vi "总磷总氮通讯.vi"() -> ()   [LabVIEW 2016, in "斯坦道总磷总氮.lvlib"]
uses:
  <vilib>/Plasmionique/MB Master/MB_Master_TCP/MB_Master_TCP.lvclass
  D:/Program Files (x86)/National Instruments/LabVIEW 2016/vi.lib/Plasmionique/MB Master/MB_Master/MB_Master.lvclass
  <vilib>/NI/Modbus Library/API/Wrapper/Create TCP Slave.vi
  <vilib>/Utility/config.llb/Write Key (Boolean).vi
  <vilib>/Utility/config.llb/Write Key (String).vi
  <vilib>/Plasmionique/MB Master/MB_Master/MB_Master.lvclass
  <vilib>/NI/Modbus Library/API/slave/Modbus Slave.lvclass
  <vilib>/Utility/config.llb/NI_LVConfig.lvlib
  <vilib>/Plasmionique/MB Master/MB Master.lvlib
  <vilib>/NI/Modbus Library/API/Wrapper/API Main.lvlib
panel:
  out "总氮测量数据区":u16[](array[numeric])
  out "总氮状态告警区":u16[](array[numeric])
  out "总磷状态告警区":u16[](array[numeric])
  out "总磷测量数据区":u16[](array[numeric])
  out "序列号":string
  out "状态告警区":T1
  out "测量数据区":T2 {"单位" items=["ug/L", "mg/L", "ppm", "mg/m3", "cm", "ppb", "ug/m3", "%", "nmol/mol", "umol/mol", "MPN/L", "MPN/100ml", "ng/m3", "NTU", "无量纲", "ms/cm", "us/cm", "℃", "mV", "万个/L"]}
  out "status":bool
  out "关键参数区":T3
  in  "读关键参数区":bool
  in  "读状态告警区":bool
  in  "读测量数据区":bool
  in  "站号":u16(ring) items=["总磷"=1, "氨氮"=3]
  in  "停止":bool
  in  "启动":bool
  in  "控制命令":u16(ring) items=["启动测量"=1, "标样核查"=2, "零点核查"=3, "跨度核查"=4, "空白测试"=5, "平行样测试"=6, "加标回收"=7, "空白校准"=8, "标样校准"=9, "初始化（清洗）"=10, "停止测试"=11, "仪器重启"=12, "校时"=13, "模式设置"=14, "测量间隔设置"=15]
  in  "控制命令参数":u16[](array[numeric]) format="%04xH"
  in  "VISA Resource":refnum<visa-resource-name>
  in  "启用模块":bool
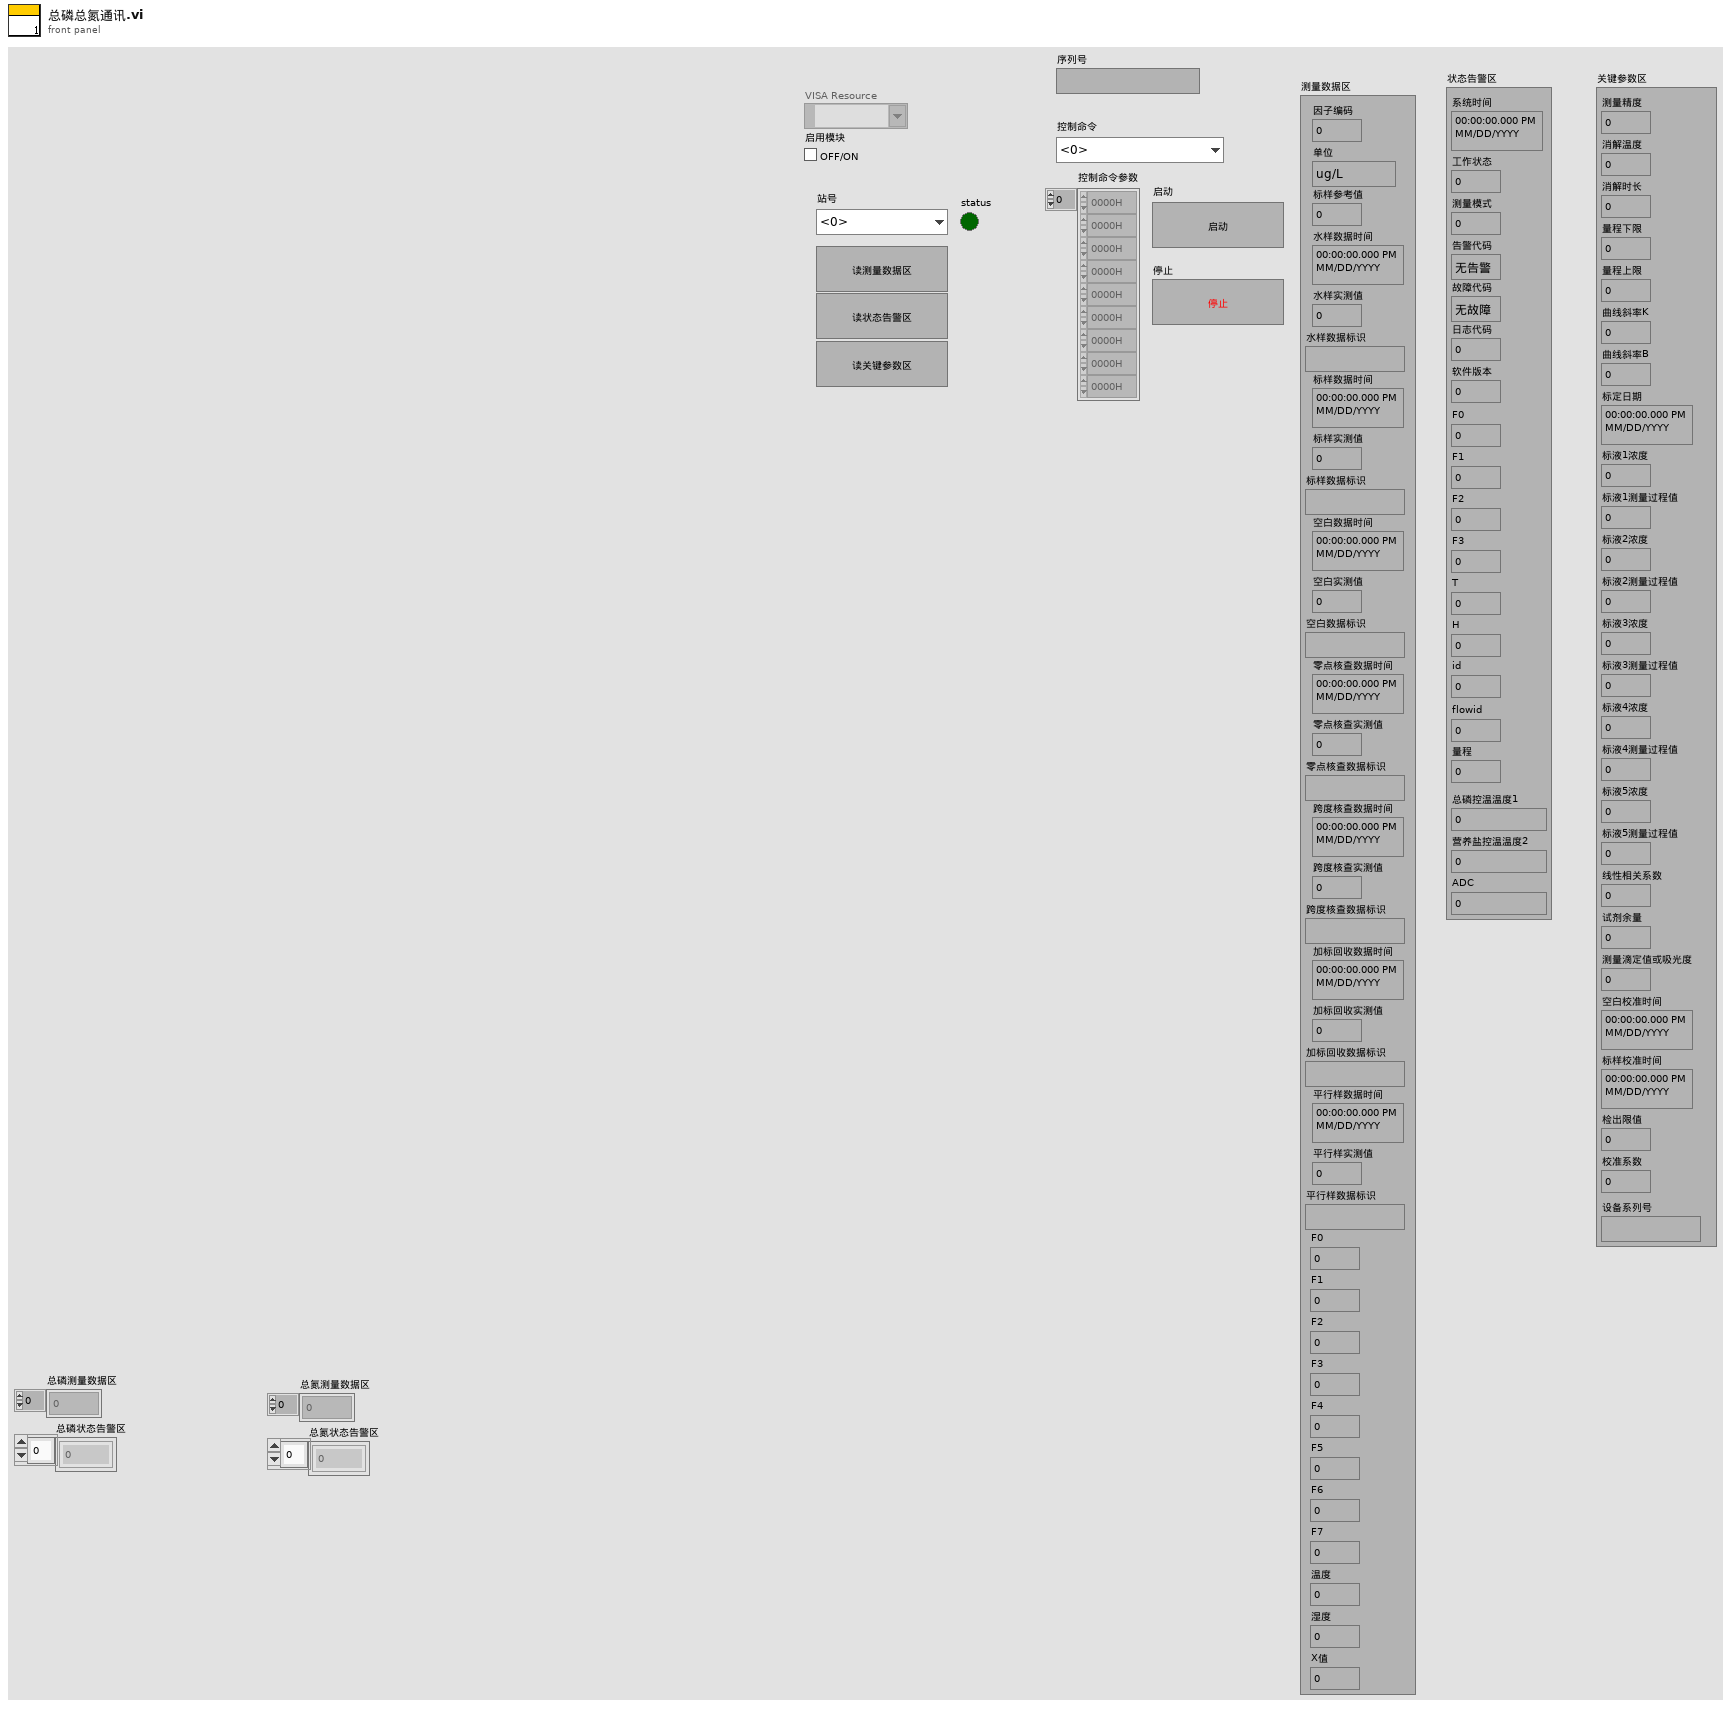
[diagram p1: front panel]
types:
  T1 = cluster{"系统时间":timestamp, "工作状态":u16, "测量模式":u16, "告警代码":enum16{"无告警", "缺试剂告警", "缺水样告警", "缺蒸馏水告警", "缺标液告警", "仪表漏液告警", "标定异常告警", "超量程告警", "加热异常", "低试剂预警", "超上限告警", "超下限告警", "仪表内部其他异常", "滴定异常告警", "电极异常告警", "量程切换告警", "参数设置告警", "PH电极电位异常", "电导率电极异常", "浊度光度异常", "溶解氧电极异常", "溶解氧光强异常", "温度异常告警", "PH异常告警", "溶解氧异常告警", "电导率异常告警", "浊度异常告警", "叶绿素异常告警", "藻密度异常告警", "蓝绿藻异常告警", "ORP异常告警", "氨氮异常告警", "清洁刷异常告警", "SD卡异常告警", "蓝牙异常告警", "Wifi异常告警", "流程异常告警"}, "故障代码":enum16{"无故障", "电机故障", "温度故障", "通讯故障", "滴定故障"}, "日志代码":u16, "软件版本":u16, "F0":sgl, "F1":sgl, "F2":sgl, "F3":sgl, "T":sgl, "H":sgl, "id":u16, "flowid":u16, "量程":u16, "总磷控温温度1":sgl, "营养盐控温温度2":sgl, "ADC":sgl}
  T2 = cluster{"因子编码":u32, "单位":u16, "标样参考值":sgl, "水样数据时间":timestamp, "水样实测值":sgl, "水样数据标识":string, "标样数据时间":timestamp, "标样实测值":sgl, "标样数据标识":string, "空白数据时间":timestamp, "空白实测值":sgl, "空白数据标识":string, "零点核查数据时间":timestamp, "零点核查实测值":sgl, "零点核查数据标识":string, "跨度核查数据时间":timestamp, "跨度核查实测值":sgl, "跨度核查数据标识":string, "加标回收数据时间":timestamp, "加标回收实测值":sgl, "加标回收数据标识":string, "平行样数据时间":timestamp, "平行样实测值":sgl, "平行样数据标识":string, "F0":sgl, "F1":sgl, "F2":sgl, "F3":sgl, "F4":sgl, "F5":sgl, "F6":sgl, "F7":sgl, "温度":sgl, "湿度":sgl, "X值":sgl}
  T3 = cluster{"测量精度":u16, "消解温度":u16, "消解时长":u16, "量程下限":sgl, "量程上限":sgl, "曲线斜率K":sgl, "曲线斜率B":sgl, "标定日期":timestamp, "标液1浓度":sgl, "标液1测量过程值":sgl, "标液2浓度":sgl, "标液2测量过程值":sgl, "标液3浓度":sgl, "标液3测量过程值":sgl, "标液4浓度":sgl, "标液4测量过程值":sgl, "标液5浓度":sgl, "标液5测量过程值":sgl, "线性相关系数":sgl, "试剂余量":u32, "测量滴定值或吸光度":sgl, "空白校准时间":timestamp, "标样校准时间":timestamp, "检出限值":sgl, "校准系数":sgl, "设备系列号":string}
  T4 = typedef "NI_LVConfig.lvlib/Config Data RefNum.ctl" = refnum<k1>
  T5 = enum8{"Enabled", "Disabled", "Disabled and Grayed Out"}
  T6 = cluster{"系统时间":timestamp, "工作状态":enum16{"空闲", "水样测试", "标样核查", "零点核查", "跨度核查", "空白测试", "平行样测试", "加标回收", "空白校准", "标样校准", "初始化（清洗）"}, "测量模式":enum16{"待机", "连续模式", "周期模式", "定点模式", "受控模式", "手动模式"}, "告警代码":enum16{"无告警", "缺试剂告警", "缺水样告警", "缺蒸馏水告警", "缺标液告警", "仪表漏液告警", "标定异常告警", "超量程告警", "加热异常", "低试剂预警", "超上限告警", "超下限告警", "仪表内部其他异常", "滴定异常告警", "电极异常告警", "量程切换告警", "参数设置告警", "PH电极电位异常", "电导率电极异常", "浊度光度异常", "溶解氧电极异常", "溶解氧光强异常", "温度异常告警", "PH异常告警", "溶解氧异常告警", "电导率异常告警", "浊度异常告警", "叶绿素异常告警", "藻密度异常告警", "蓝绿藻异常告警", "ORP异常告警", "氨氮异常告警", "清洁刷异常告警", "SD卡异常告警", "蓝牙异常告警", "Wifi异常告警", "流程异常告警"}, "故障代码":enum16{"无故障", "电机故障", "温度故障", "通讯故障", "滴定故障"}, "日志代码":u16, "软件版本":u16, "F0":sgl, "F1":sgl, "F2":sgl, "F3":sgl, "T":sgl, "H":sgl, "id":u16, "flowid":u16, "量程":u16, "总磷控温温度1":sgl, "营养盐控温温度2":sgl, "ADC":sgl}
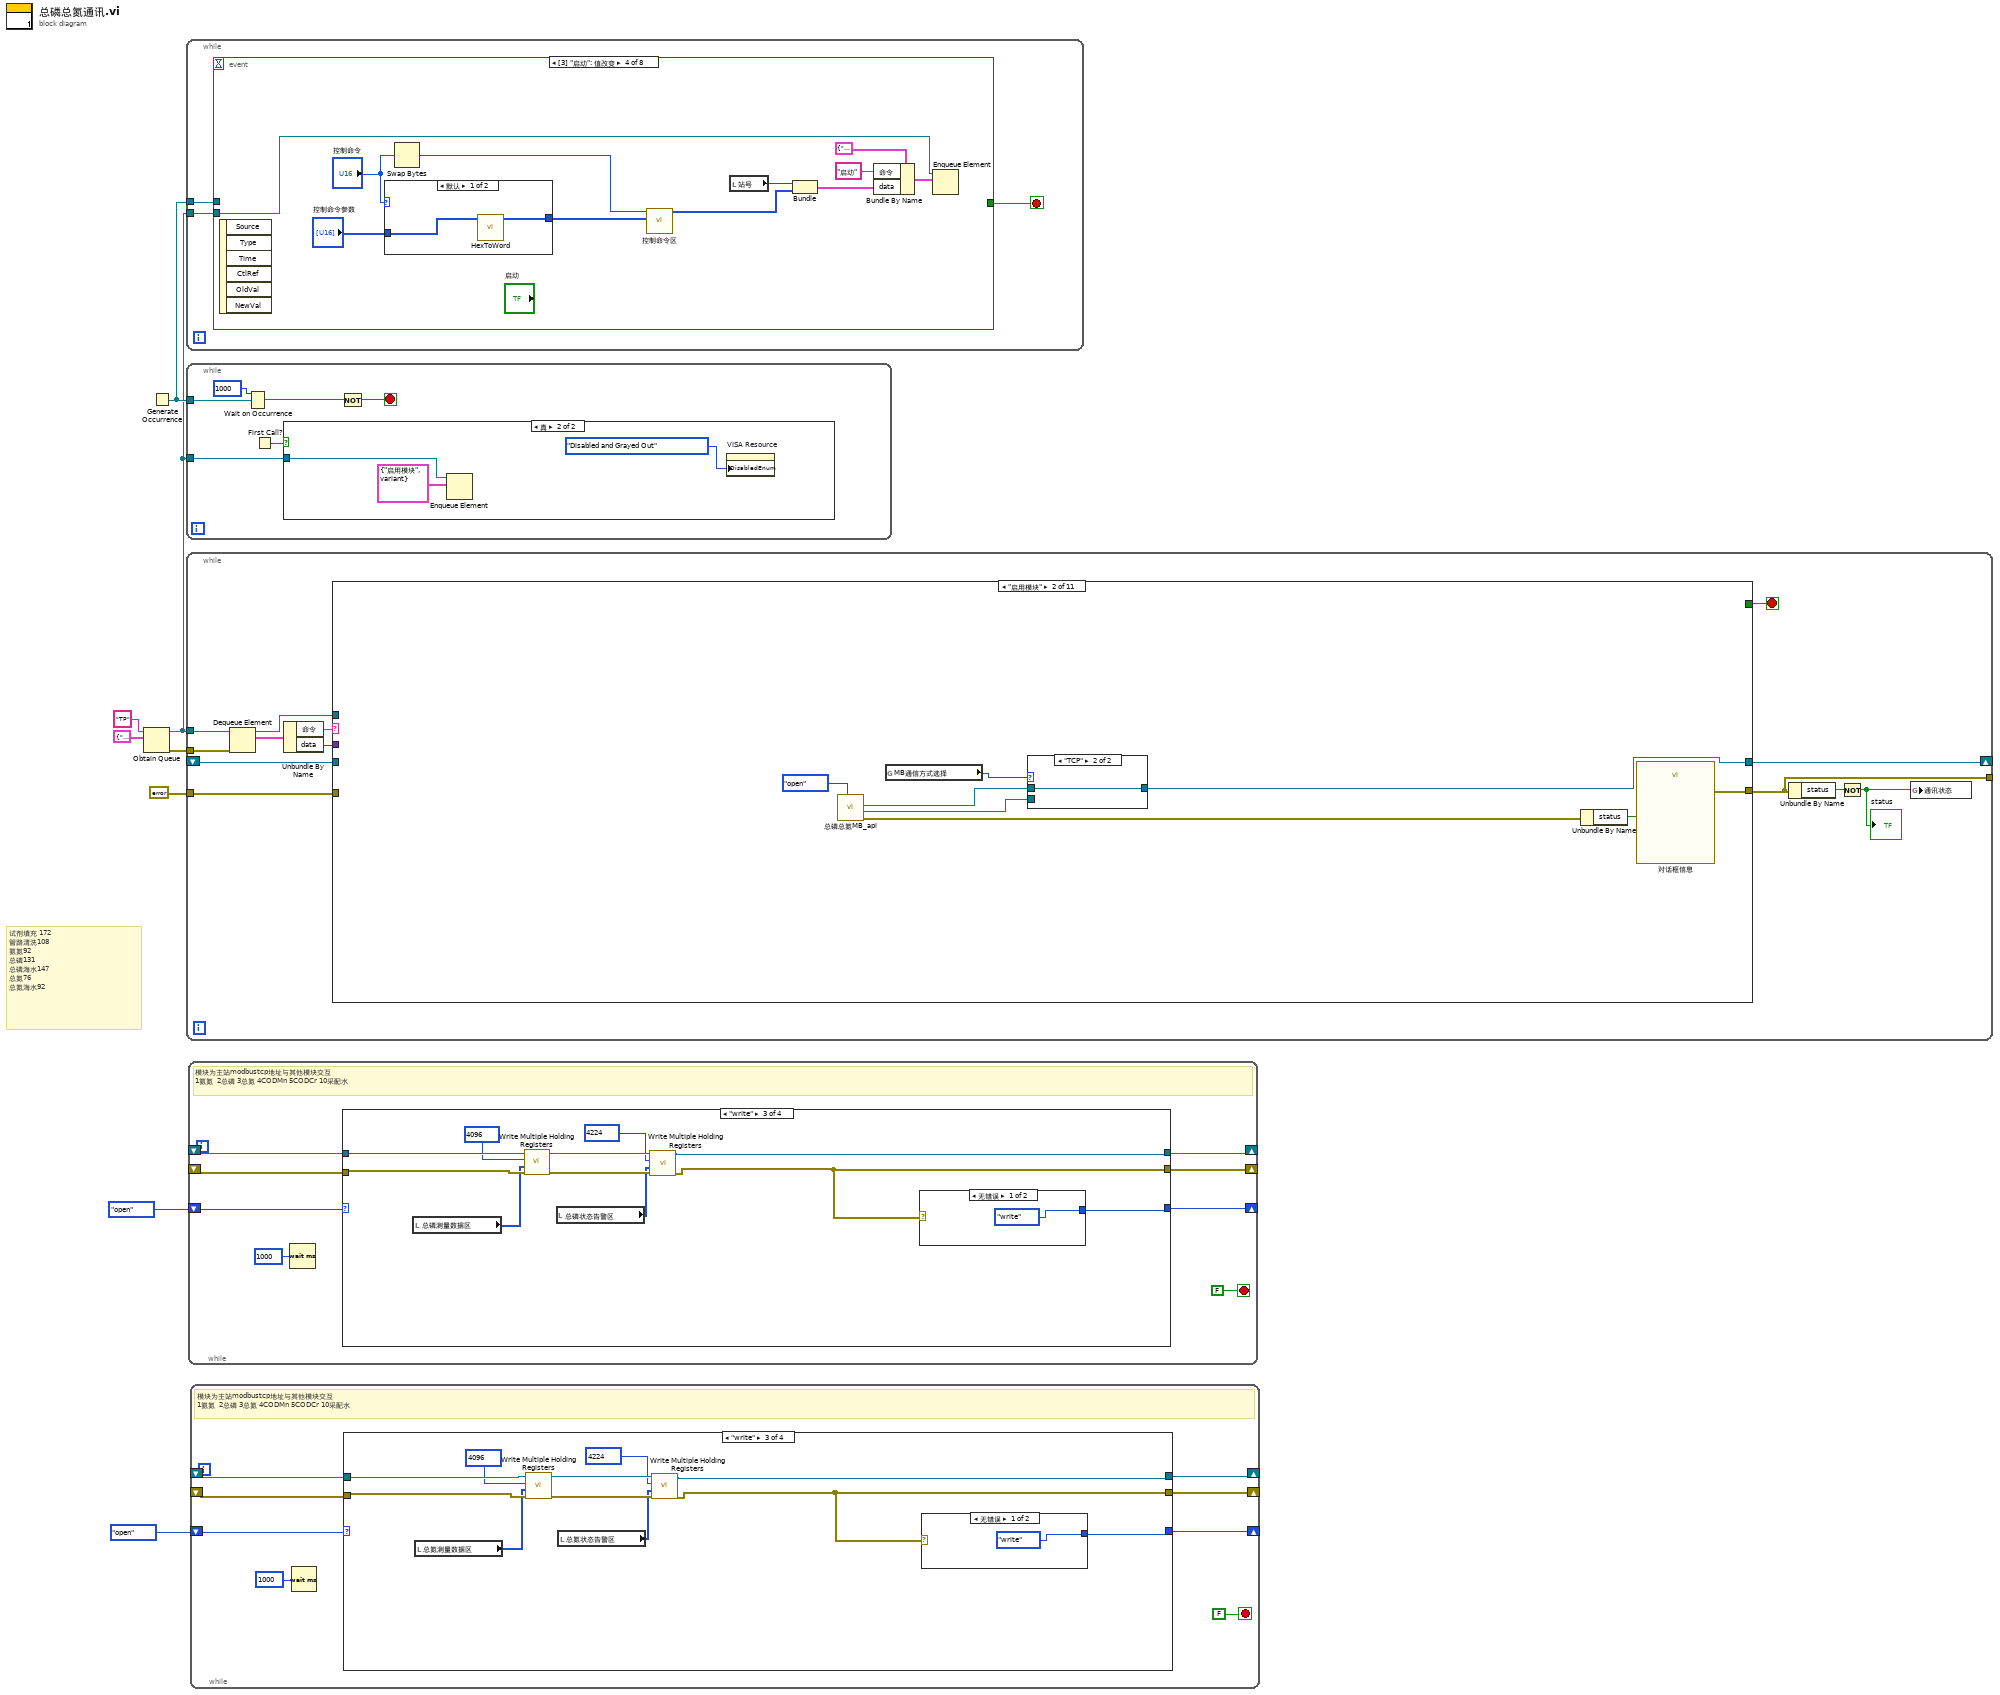
[diagram p0: block diagram]
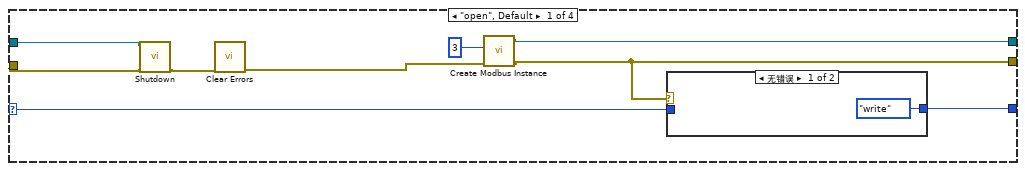
[diagram p2: hidden frame]
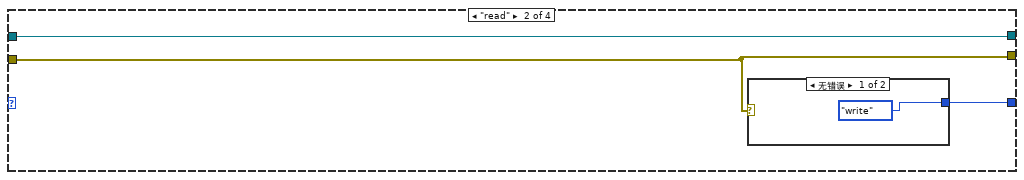
[diagram p4: hidden frame]
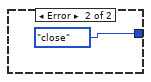
[diagram p5: hidden frame]
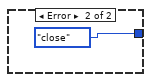
[diagram p6: hidden frame]
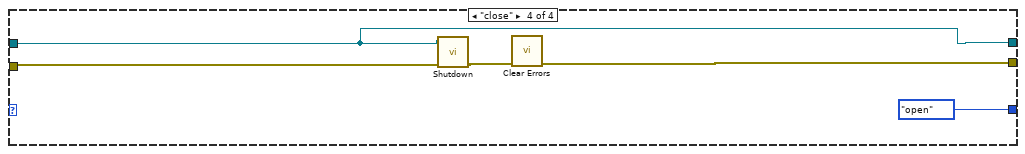
[diagram p7: hidden frame]
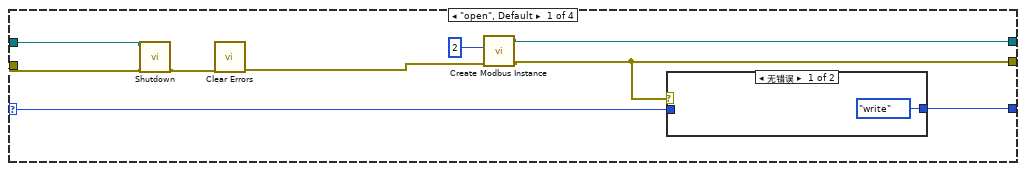
[diagram p8: hidden frame]
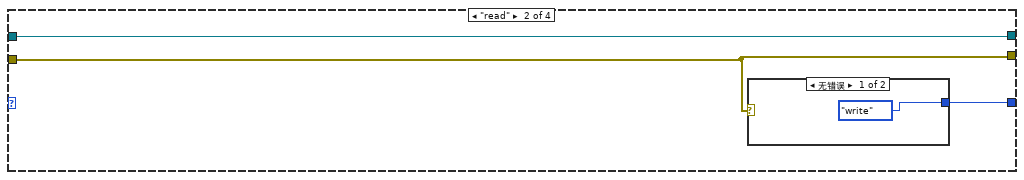
[diagram p10: hidden frame]
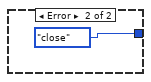
[diagram p11: hidden frame]
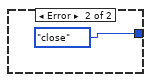
[diagram p12: hidden frame]
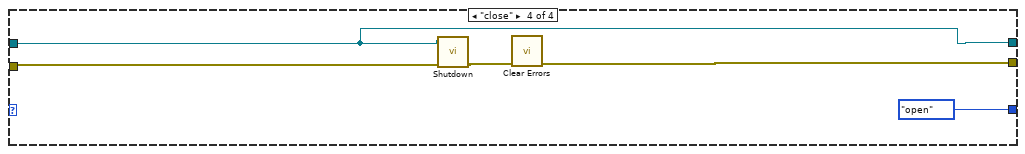
[diagram p13: hidden frame]
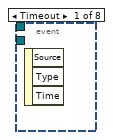
[diagram p15: hidden frame]
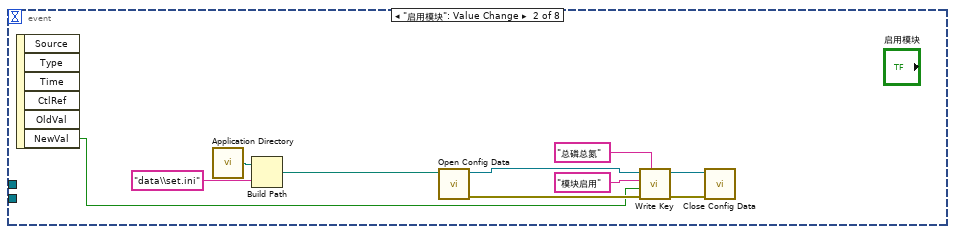
[diagram p16: hidden frame]
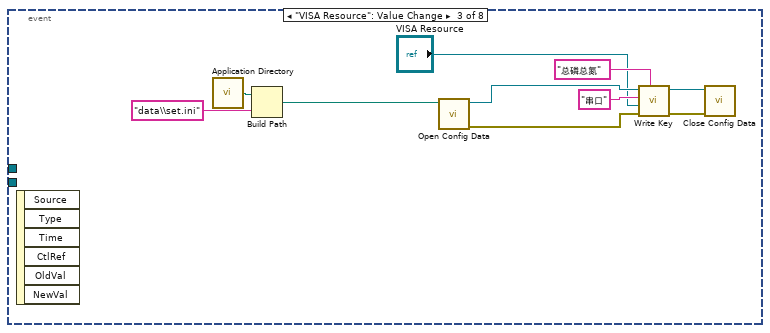
[diagram p17: hidden frame]
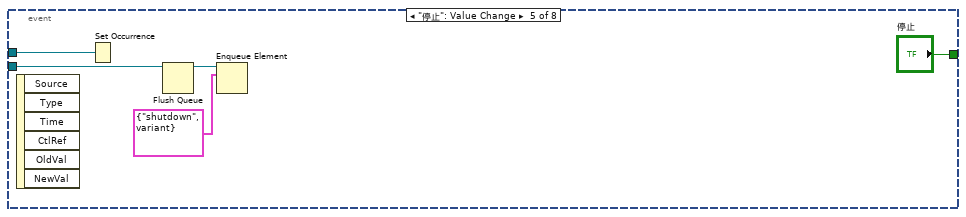
[diagram p19: hidden frame]
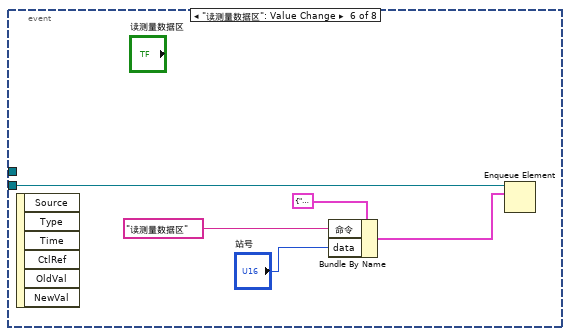
[diagram p20: hidden frame]
diagram:
  # "试剂填充 172 \n管路清洗108\n氨氮92\n总磷131\n总磷海水147\n总氮76\n总氮海水92"
  n1 = Obtain Queue(name (unnamed)="TP" ("名称（未命名）"), element data type=cluster{"命令":string, "data":variant} {"命令"="", "data"=variant}) -> (queue out=w3:refnum<queue>, error out=w6:errorcluster)  [unwired: 3 in, 1 out]
  n2 = Generate Occurrence() -> (w4:refnum<k4>)
  n3 = while {
    tunnel: w3 -> [w11]
    tunnel: w4 -> [w9]
    stop <- w10 stop-if-true
    n4 = event shown="[3] \"启动\": 值改变" {
      selector: _ -> [_ _ _ _ _ _ _ _]
      dyn-events: _ -> [_ _ _ _ _ _ _ _]
      timeout: _ -> [_ _ _ _ _ _ _ _]
      tunnel: w11 -> [_ _ _ w42 w49 w55 w60 w65]
      tunnel: [_ _ _ _ "停止" _ _ _] -> w10
      tunnel: w9 -> [_ _ _ _ w46 _ _ _]
      event Timeout {
        n5 = event-data() -> ()  [unwired: 1 in, 3 out]
      }
      event "启用模块": Value Change {
        n6 = event-data() -> ("NewVal"=w12:bool)  [unwired: 1 in, 5 out]
        n7 = call <vilib>:"Application Directory.vi"() -> ("Application Directory"=w14:path)
        n8 = Build Path(base path=w14, name or relative path="data\\set.ini" ("名称或相对路径")) -> (appended path=w15:path)
        n9 = call <vilib>:"Open Config Data.vi"("configuration file path"=w15) -> ("error out"=w21:errorcluster, "refnum"=w20:T4)  [unwired: 8 in, 1 out]
        n10 = call-poly <vilib>:"Write Key.vi"("section"="总磷总氮", "error in (no error)"=w21, "value"=w12, "key"="模块启用", "refnum"=w20) -> ("error out"=w17:errorcluster, "refnum out"=w13:T4)  [unwired: 4 in, 1 out]
        n11 = call <vilib>:"Close Config Data.vi"("error in (no error)"=w17, "refnum"=w13) -> ()  [unwired: 8 in, 2 out]
      }
      event "VISA Resource": Value Change {
        n12 = event-data() -> ()  [unwired: 1 in, 6 out]
        n13 = call <vilib>:"Application Directory.vi"() -> ("Application Directory"=w24:path)
        n14 = Build Path(base path=w24, name or relative path="data\\set.ini" ("名称或相对路径")) -> (appended path=w25:path)
        n15 = call <vilib>:"Open Config Data.vi"("configuration file path"=w25) -> ("error out"=w31:errorcluster, "refnum"=w30:T4)  [unwired: 8 in, 1 out]
        n16 = call-poly <vilib>:"Write Key.vi"("section"="总磷总氮", "error in (no error)"=w31, "value"="VISA Resource", "key"="串口", "refnum"=w30) -> ("error out"=w27:errorcluster, "refnum out"=w23:T4)  [unwired: 4 in, 1 out]
        n17 = call <vilib>:"Close Config Data.vi"("error in (no error)"=w27, "refnum"=w23) -> ()  [unwired: 8 in, 2 out]
      }
      event "启动": Value Change {
        n18 = event-data() -> ()  [unwired: 1 in, 6 out]
        n19 = case shown="默认" "控制命令" {
          tunnel: "控制命令参数" -> [w44 w45]
          tunnel: [w43 w45] -> w32
          frame Default {
            n20 = call "HexToWord.vi"("数组"=w44) -> ("WORD"=w43:u16[])  [unwired: 10 in]
          }
          frame 13 {
          }
        }
        n21 = Swap Bytes(anything="控制命令") -> (byte swapped=w35:u16)
        n22 = call "控制命令区.vi"("控制命令参数"=w32, "控制命令"=w35) -> ("控制命令"=w38:u16[])  [unwired: 9 in]
        n23 = local read "站号"() -> (w37:u16)
        n24 = Bundle("站号"=w37, "控制命令"=w38) -> (w36:cluster{"站号":u16, "控制命令":u16[]})  [unwired: 1 in]
        n25 = Bundle By Name(cluster=cluster{"命令":string, "data":variant} {"命令"="", "data"=variant} ("元素"), "命令"="启动", "data"=w36) -> (w40:cluster{"命令":string, "data":variant})
        n26 = Enqueue Element(queue=w42, element=w40) -> ()  [unwired: 2 in, 3 out]
      }
      event "停止": Value Change {
        n27 = event-data() -> ()  [unwired: 1 in, 6 out]
        n28 = Set Occurrence(w46) -> ()
        n29 = Flush Queue(queue=w49) -> (queue out=w48:refnum<queue>)  [unwired: 1 in, 2 out]
        n30 = Enqueue Element(queue=w48, element=cluster{"命令":string, "data":variant} {"命令"="shutdown", "data"=variant} ("元素")) -> ()  [unwired: 2 in, 3 out]
      }
      event "读测量数据区": Value Change {
        n31 = event-data() -> ()  [unwired: 1 in, 6 out]
        n32 = Bundle By Name(cluster=cluster{"命令":string, "data":variant} {"命令"="", "data"=variant} ("元素"), "命令"="读测量数据区", "data"="站号") -> (w53:cluster{"命令":string, "data":variant})
        n33 = Enqueue Element(queue=w55, element=w53) -> ()  [unwired: 2 in, 3 out]
      }
      event "读状态告警区": Value Change {
        n34 = event-data() -> ()  [unwired: 1 in, 6 out]
        n35 = local read "站号"() -> (w56:u16)
        n36 = Bundle By Name(cluster=cluster{"命令":string, "data":variant} {"命令"="", "data"=variant} ("元素"), "命令"="读状态告警区", "data"=w56) -> (w58:cluster{"命令":string, "data":variant})
        n37 = Enqueue Element(queue=w60, element=w58) -> ()  [unwired: 2 in, 3 out]
      }
      event "读关键参数区": Value Change {
        n38 = event-data() -> ()  [unwired: 1 in, 6 out]
        n39 = local read "站号"() -> (w61:u16)
        n40 = Bundle By Name(cluster=cluster{"命令":string, "data":variant} {"命令"="", "data"=variant} ("元素"), "命令"="读关键参数区", "data"=w61) -> (w63:cluster{"命令":string, "data":variant})
        n41 = Enqueue Element(queue=w65, element=w63) -> ()  [unwired: 2 in, 3 out]
      }
    }
  }
  n42 = while {
    tunnel: w4 -> [w71]
    tunnel: w3 -> [w67]
    stop <- w68 stop-if-true
    n43 = Wait on Occurrence(2:w71, 3:1000 ("毫秒超时(-1)")) -> (0:w69:bool)  [unwired: 1 in]
    n44 = First Call?() -> (First Call?: T/F=w66:bool)
    n45 = case shown="真" w66 {
      tunnel: w67 -> [_ w73]
      frame False {
      }
      frame True {
        n46 = Enqueue Element(queue=w73, element=cluster{"命令":string, "data":variant} {"命令"="启用模块", "data"=variant} ("元素")) -> ()  [unwired: 2 in, 3 out]
        n47 = property on="VISA Resource" class="VISAName"("DisabledEnum"=T5."Disabled and Grayed Out" ("禁用")) -> ()  [unwired: 2 in, 2 out]
      }
    }
    n48 = Not(x=w69) -> (.not. x?=w68:bool)
  }
  n49 = while {
    tunnel: w3 -> [w87]
    tunnel: w6 -> [w86]
    shift-right: [w84] -> _
    shift-left: _ -> [w83]
    tunnel: errorcluster {"status"=FALSE, "code"=0, "source"=""} ("error out") -> [w82]
    tunnel: [w77] -> _
    stop <- w85 stop-if-true
    n50 = Dequeue Element(queue=w87, error in (no error)=w86) -> (queue out=w78:refnum<queue>, element=w80:cluster{"命令":string, "data":variant})  [unwired: 1 in, 2 out]
    n51 = Unbundle By Name(w80) -> ("命令"=w81:string, "data"=w79:variant)
    n52 = case shown="\"启用模块\"" w81 {
      tunnel: w79 -> [_ _ _ w113 w124 w141 w151 w205 w223 w237 _]
      tunnel: w78 -> [_ _ _ _ _ _ _ _ _ _ w250]
      tunnel: [_ _ _ _ _ _ _ _ _ _ TRUE] -> w85
      tunnel: [w88 w90 w100 w116 w127 w143 w155 w214 w230 w244 w246] -> w84
      tunnel: [w89 w96 w101 w115 w126 w142 w156 w204 w231 w245 w247] -> w77
      tunnel: w83 -> [w88 _ w100 w112 w123 w140 w150 w208 w226 w240 w246]
      tunnel: w82 -> [w89 _ w103 w109 w120 w137 w148 w209 w227 w241 w248]
      frame Default {
      }
      frame "启用模块" {
        n53 = call "总磷总氮MB_api.vi"("STEP"=enum16{"open", "read", "write", "close"}."open") -> ("error out"=w94:errorcluster, "MB session out"=w91:refnum<class "MB_Master.lvclass">, "MB_TCP session"=w92:refnum<class "MB_Master_TCP.lvclass">)  [unwired: 7 in, 1 out]
        n54 = global read "总磷总氮断电保存全局变量.vi" "MB通信方式选择"() -> (w93:enum16{"串口", "TCP"})
        n55 = case shown="\"TCP\"" w93 {
          tunnel: w92 -> [_ w99]
          tunnel: w91 -> [w98 _]
          tunnel: [w98 w99] -> w90
          frame "串口", Default {
          }
          frame "TCP" {
          }
        }
        n56 = Unbundle By Name(w94) -> ("status"=w97:bool)
        n57 = call "对话框信息"("Enable"=w97) -> ("error out"=w96:errorcluster)  [unwired: 9 in, 1 out]
      }
      frame "停用模块" {
        n58 = call-dynamic "Close Session.vi"("error in (no error)"=w103, "MB session in"=w100) -> ("error out"=w102:errorcluster)  [unwired: 9 in]
        n59 = call <vilib>:"Clear Errors.vi"("error in (no error)"=w102) -> ("error out"=w101:errorcluster)  [unwired: 5 in, 1 out]
      }
      frame "启动" {
        n60 = Variant To Data(type=cluster{"站号":u16, "控制命令":u16[]} {"站号"=0, "控制命令"=[]} ("输出簇"), Variant=w113) -> (data=w107:cluster{"站号":u16, "控制命令":u16[]})  [unwired: 1 in, 1 out]
        n61 = Unbundle By Name(w107) -> ("站号"=w106:u16, "控制命令"=w104:u16[])
        n62 = property class="MB_Master"(reference=w112, error in=w109, "Properties:Slave ID"=w106) -> (reference out=w111:refnum<class "MB_Master.lvclass">, error out=w110:errorcluster)
        n63 = Index Array(array=w104) -> (element=w105:u16)  [unwired: 1 in]
        n64 = global write "VAR总磷总氮全局变量.vi" "控制命令"(w105) -> ()
        n65 = call <vilib>:"Write Multiple Registers.vi"("error in (no error)"=w110, "values"=w104, "starting address"=u16 4608, "MB session in"=w111) -> ("error out"=w115:errorcluster, "MB session out"=w116:refnum<class "MB_Master.lvclass">)  [unwired: 6 in]
      }
      frame "盲样测试" {
        n66 = Variant To Data(type=0, Variant=w124) -> (data=w117:i32)  [unwired: 1 in, 1 out]
        n67 = case shown="默认" w117 {
          tunnel: [u16[] [] ("values") u16[] [33539, 0] ("values") u16[] [23555, 0] ("values")] -> w119
          frame Default {
          }
          frame 1 {
            # "总磷盲样测试命令"
          }
          frame 3 {
            # "氨氮盲样测试"
          }
        }
        n68 = property class="MB_Master"(reference=w123, error in=w120, "Properties:Slave ID"=w117) -> (reference out=w122:refnum<class "MB_Master.lvclass">, error out=w121:errorcluster)
        n69 = call <vilib>:"Write Multiple Registers.vi"("error in (no error)"=w121, "values"=w119, "starting address"=u16 24592, "MB session in"=w122) -> ("error out"=w126:errorcluster, "MB session out"=w127:refnum<class "MB_Master.lvclass">)  [unwired: 6 in]
      }
      frame "debug" {
        n70 = Variant To Data(type=cluster{"站号":u16, "控制命令":u16[]} {"站号"=0, "控制命令"=[]} ("输出簇"), Variant=w141) -> (data=w135:cluster{"站号":u16, "控制命令":u16[]})  [unwired: 1 in, 1 out]
        n71 = Unbundle By Name(w135) -> ("站号"=w134:u16, "控制命令"=w132:u16[])
        n72 = property class="MB_Master"(reference=w140, error in=w137, "Properties:Slave ID"=w134) -> (reference out=w139:refnum<class "MB_Master.lvclass">, error out=w138:errorcluster)
        n73 = Index Array(array=w132) -> (element=w133:u16)  [unwired: 1 in]
        n74 = global write "VAR总磷总氮全局变量.vi" "控制命令"(w133) -> ()
        n75 = call <vilib>:"Write Multiple Registers.vi"("error in (no error)"=w138, "values"=w132, "starting address"=u16 24594, "MB session in"=w139) -> ("error out"=w142:errorcluster, "MB session out"=w143:refnum<class "MB_Master.lvclass">)  [unwired: 6 in]
      }
      frame "读测量数据区" {
        n76 = Variant To Data(type=u8 1 ("Slave ID"), Variant=w151) -> (data=w146:u8)  [unwired: 1 in, 1 out]
        n77 = property class="MB_Master"(reference=w150, error in=w148, "Properties:Slave ID"=w146) -> (reference out=w149:refnum<class "MB_Master.lvclass">, error out=w147:errorcluster)
        n78 = call <vilib>:"Read Holding Registers.vi"("error in (no error)"=w147, "quantity"=u16 104, "starting address"=u16 4096, "MB session in"=w149) -> ("error out"=w156:errorcluster, "Registers"=w144:u16[], "MB session out"=w155:refnum<class "MB_Master.lvclass">)  [unwired: 5 in]
        n79 = call "测量数据区.vi"("数组"=w144) -> ("测量数据区"=w145:T2)  [unwired: 10 in]
        "测量数据区" <- w145
        n80 = global write "VAR总磷总氮全局变量.vi" "测量数据区"(w145) -> ()
        n81 = case shown="2" w146 {
          tunnel: w145 -> [_ w198 w200]
          tunnel: w144 -> [_ w157 w199]
          frame 0, Default {
          }
          frame 1 {
            n82 = global read "VAR总磷总氮全局变量.vi" "总磷状态告警区"() -> (w167:T6)
            n83 = global read "VAR总磷总氮全局变量.vi" "总氮状态告警区"() -> (w166:T6)
            n84 = global read "VAR总磷总氮全局变量.vi" "总氮状态告警区"() -> (w178:T6)
            n85 = global read "VAR总磷总氮全局变量.vi" "总磷状态告警区"() -> (w177:T6)
            n86 = Unbundle By Name(w167) -> ("量程"=w163:u16)
            n87 = Unbundle By Name(w166) -> ("量程"=w165:u16)
            n88 = Unbundle By Name(w178) -> ("量程"=w176:u16)
            n89 = Unbundle By Name(w177) -> ("量程"=w175:u16)
            n90 = Equal To 0?(x=w163) -> (x = 0?=w168:bool)
            n91 = global read "总磷总氮断电保存全局变量.vi" "总氮稀释倍数"() -> (w158:dbl)
            n92 = global read "总磷总氮断电保存全局变量.vi" "总氮稀释倍数"() -> (w159:dbl)
            n93 = Equal?(x=w165, y=u16 1) -> (x = y?=w169:bool)
            n94 = And(x=w169, y=w168) -> (x .and. y?=w162:bool)
            n95 = Equal To 0?(x=w176) -> (x = 0?=w172:bool)
            n96 = Equal?(x=w175, y=u16 1) -> (x = y?=w173:bool)
            n97 = And(x=w172, y=w173) -> (x .and. y?=w171:bool)
            n98 = Reciprocal(x=w158) -> (1/x=w170:dbl)
            n99 = Select(t=w159, s=w162, f=1.0) -> (s? t:f=w160:dbl)
            n100 = Unbundle By Name(w198) -> ("水样实测值"=w197:sgl, "标样实测值"=w195:sgl, "空白实测值"=w193:sgl, "零点核查实测值"=w191:sgl, "跨度核查实测值"=w189:sgl, "加标回收实测值"=w187:sgl, "平行样实测值"=w185:sgl)
            n101 = Select(t=w170, s=w171, f=w160) -> (s? t:f=w183:dbl)
            n102 = Multiply(x=w197, y=w183) -> (x*y=w196:dbl)
            n103 = Multiply(x=w195, y=w183) -> (x*y=w194:dbl)
            n104 = Multiply(x=w193, y=w183) -> (x*y=w192:dbl)
            n105 = Multiply(x=w191, y=w183) -> (x*y=w190:dbl)
            n106 = Multiply(x=w189, y=w183) -> (x*y=w188:dbl)
            n107 = Multiply(x=w187, y=w183) -> (x*y=w186:dbl)
            n108 = Multiply(x=w185, y=w183) -> (x*y=w184:dbl)
            n109 = global read "VAR总磷总氮全局变量.vi" "总氮测量数据区"() -> (w181:T2)
            n110 = global read "VAR总磷总氮全局变量.vi" "总磷测量数据区"() -> (w179:T2)
            n111 = Bundle By Name(cluster=w198, "水样实测值"=w196, "标样实测值"=w194, "空白实测值"=w192, "零点核查实测值"=w190, "跨度核查实测值"=w188, "加标回收实测值"=w186, "平行样实测值"=w184) -> (w182:T2)
            n112 = call "总磷数据时间处理.vi"("总磷修正数据输入"=w179, "总氮原始数据"=w181, "总磷原始数据"=w182) -> ("总磷修正数据输出"=w180:T2)  [unwired: 8 in]
            n113 = global write "VAR总磷总氮全局变量.vi" "总磷测量数据区"(w180) -> ()
            "总磷测量数据区" <- w157
          }
          frame 2 {
            n114 = global write "VAR总磷总氮全局变量.vi" "总氮测量数据区"(w200) -> ()
            "总氮测量数据区" <- w199
          }
        }
      }
      frame "读状态告警区" {
        n115 = Variant To Data(type=u8 1 ("Slave ID"), Variant=w205) -> (data=w210:u8)  [unwired: 1 in, 1 out]
        n116 = property class="MB_Master"(reference=w208, error in=w209, "Properties:Slave ID"=w210) -> (reference out=w207:refnum<class "MB_Master.lvclass">, error out=w206:errorcluster)
        n117 = call <vilib>:"Read Holding Registers.vi"("error in (no error)"=w206, "quantity"=u16 29, "starting address"=u16 4224, "MB session in"=w207) -> ("error out"=w204:errorcluster, "Registers"=w201:u16[], "MB session out"=w214:refnum<class "MB_Master.lvclass">)  [unwired: 5 in]
        n118 = call "状态告警区.vi"("数组"=w201) -> ("状态告警区"=w202:T6)  [unwired: 10 in]
        "状态告警区" <- w202
        n119 = global write "VAR总磷总氮全局变量.vi" "状态告警区"(w202) -> ()
        n120 = Unbundle By Name(w202) -> ("id"=w203:u16)
        n121 = case shown="1, 131" w203 {
          tunnel: w202 -> [_ w216 w218]
          tunnel: w201 -> [_ w215 w217]
          frame 0, Default {
          }
          frame 1, 131 {
            n122 = global write "VAR总磷总氮全局变量.vi" "总磷状态告警区"(w216) -> ()
            "总磷状态告警区" <- w215
          }
          frame 2, 76 {
            n123 = global write "VAR总磷总氮全局变量.vi" "总氮状态告警区"(w218) -> ()
            "总氮状态告警区" <- w217
          }
        }
      }
      frame "读关键参数区" {
        n124 = Variant To Data(type=u8 1 ("Slave ID"), Variant=w223) -> (data=w221:u8)  [unwired: 1 in, 1 out]
        n125 = property class="MB_Master"(reference=w226, error in=w227, "Properties:Slave ID"=w221) -> (reference out=w225:refnum<class "MB_Master.lvclass">, error out=w224:errorcluster)
        n126 = call <vilib>:"Read Holding Registers.vi"("error in (no error)"=w224, "quantity"=u16 19, "starting address"=u16 4256, "MB session in"=w225) -> ("error out"=w231:errorcluster, "Registers"=w220:u16[], "MB session out"=w230:refnum<class "MB_Master.lvclass">)  [unwired: 5 in]
        n127 = call "关键参数区.vi"("数组"=w220) -> ("关键参数区"=w219:T3)  [unwired: 10 in]
        "关键参数区" <- w219
        n128 = global write "VAR总磷总氮全局变量.vi" "关键参数区"(w219) -> ()
      }
      frame "读序列号" {
        n129 = Variant To Data(type=u8 1 ("Slave ID"), Variant=w237) -> (data=w235:u8)  [unwired: 1 in, 1 out]
        n130 = property class="MB_Master"(reference=w240, error in=w241, "Properties:Slave ID"=w235) -> (reference out=w239:refnum<class "MB_Master.lvclass">, error out=w238:errorcluster)
        n131 = call <vilib>:"Read Holding Registers.vi"("error in (no error)"=w238, "quantity"=u16 6, "starting address"=u16 3, "MB session in"=w239) -> ("error out"=w245:errorcluster, "Registers"=w234:u16[], "MB session out"=w244:refnum<class "MB_Master.lvclass">)  [unwired: 5 in]
        n132 = call "HexToString.vi"("数组"=w234) -> ("STRING"=w233:string[])  [unwired: 10 in]
        n133 = Index Array(array=w233) -> (element=w232:string)  [unwired: 1 in]
        "序列号" <- w232
        n134 = global write "VAR总磷总氮全局变量.vi" "序列号"(w232) -> ()
      }
      frame "shutdown" {
        n135 = call-dynamic "Close Session.vi"("error in (no error)"=w248, "MB session in"=w246) -> ("error out"=w247:errorcluster)  [unwired: 9 in]
        n136 = Flush Queue(queue=w250) -> (queue out=w249:refnum<queue>)  [unwired: 1 in, 2 out]
        n137 = Release Queue(queue=w249) -> ()  [unwired: 2 in, 3 out]
      }
    }
    n138 = Unbundle By Name(w77) -> ("status"=w76:bool)
    n139 = Not(x=w76) -> (.not. x?=w75:bool)
    "status" <- w75
    n140 = global write "VAR总磷总氮全局变量.vi" "通讯状态"(w75) -> ()
  }
  n141 = while {
    shift-right: [w257] -> _
    shift-left: _ -> [w259]
    shift-right: [w256] -> _
    shift-left: _ -> [w258]
    shift-right: [w253] -> _
    shift-left: enum16{"open", "read", "write", "close"}."open" -> [w254]
    stop <- FALSE stop-if-true
    # "模块为主站modbustcp地址与其他模块交互\n1氨氮  2总磷 3总氮 4CODMn 5CODCr 10采配水"
    n142 = Wait (ms)(milliseconds to wait=u32 1000 ("等待时间（毫秒）")) -> ()  [unwired: 1 out]
    n143 = case shown="\"write\"" w254 {
      selector: w254 -> [w268 _ _ _]
      tunnel: w259 -> [w262 w271 w285 w291]
      tunnel: w258 -> [w261 w272 w284 w290]
      tunnel: [w265 w271 w280 w291] -> w257
      tunnel: [w264 w272 w279 w293] -> w256
      tunnel: [w267 w273 w286 enum16{"open", "read", "write", "close"}."open"] -> w253
      frame "open", Default {
        n144 = call-dynamic "Shutdown.vi"("error in"=w261, "Modbus slave in"=w262) -> ("error out"=w260:errorcluster)  [unwired: 9 in]
        n145 = call <vilib>:"Clear Errors.vi"("error in (no error)"=w260) -> ("error out"=w263:errorcluster)  [unwired: 5 in, 1 out]
        n146 = call-poly <vilib>:"Create Modbus Instance.vi"("error in"=w263, "port (502)"=u16 2) -> ("error out"=w264:errorcluster, "TCP slave instance"=w265:refnum<class "Modbus Slave.lvclass">)  [unwired: 8 in]
        n147 = case shown="无错误" w264 {
          tunnel: w268 -> [_ w270]
          tunnel: [enum16{"open", "read", "write", "close"}."write" w270] -> w267
          frame No Error {
          }
          frame Error {
          }
        }
      }
      frame "read" {
        n148 = case shown="无错误" w272 {
          tunnel: [enum16{"open", "read", "write", "close"}."write" enum16{"open", "read", "write", "close"}."close"] -> w273
          frame No Error {
          }
          frame Error {
          }
        }
      }
      frame "write" {
        n149 = local read "总磷测量数据区"() -> (w278:u16[])
        n150 = call-dynamic "Write Multiple Holding Registers.vi"("error in"=w284, "registers to write"=w278, "starting address"=u16 4096, "Modbus slave in"=w285) -> ("error out"=w281:errorcluster, "Modbus slave out"=w282:refnum<class "Modbus Slave.lvclass">)  [unwired: 6 in]
        n151 = local read "总磷状态告警区"() -> (w276:u16[])
        n152 = call-dynamic "Write Multiple Holding Registers.vi"("error in"=w281, "registers to write"=w276, "starting address"=u16 4224, "Modbus slave in"=w282) -> ("error out"=w279:errorcluster, "Modbus slave out"=w280:refnum<class "Modbus Slave.lvclass">)  [unwired: 6 in]
        n153 = case shown="无错误" w279 {
          tunnel: [enum16{"open", "read", "write", "close"}."write" enum16{"open", "read", "write", "close"}."close"] -> w286
          frame No Error {
          }
          frame Error {
          }
        }
      }
      frame "close" {
        n154 = call-dynamic "Shutdown.vi"("error in"=w290, "Modbus slave in"=w291) -> ("error out"=w289:errorcluster)  [unwired: 9 in]
        n155 = call <vilib>:"Clear Errors.vi"("error in (no error)"=w289) -> ("error out"=w293:errorcluster)  [unwired: 5 in, 1 out]
      }
    }
  }
  n156 = while {
    shift-right: [w299] -> _
    shift-left: _ -> [w301]
    shift-right: [w298] -> _
    shift-left: _ -> [w300]
    shift-right: [w295] -> _
    shift-left: enum16{"open", "read", "write", "close"}."open" -> [w296]
    stop <- FALSE stop-if-true
    # "模块为主站modbustcp地址与其他模块交互\n1氨氮  2总磷 3总氮 4CODMn 5CODCr 10采配水"
    n157 = Wait (ms)(milliseconds to wait=u32 1000 ("等待时间（毫秒）")) -> ()  [unwired: 1 out]
    n158 = case shown="\"write\"" w296 {
      selector: w296 -> [w310 _ _ _]
      tunnel: w301 -> [w304 w313 w327 w333]
      tunnel: w300 -> [w303 w314 w326 w332]
      tunnel: [w307 w313 w322 w333] -> w299
      tunnel: [w306 w314 w321 w335] -> w298
      tunnel: [w309 w315 w328 enum16{"open", "read", "write", "close"}."open"] -> w295
      frame "open", Default {
        n159 = call-dynamic "Shutdown.vi"("error in"=w303, "Modbus slave in"=w304) -> ("error out"=w302:errorcluster)  [unwired: 9 in]
        n160 = call <vilib>:"Clear Errors.vi"("error in (no error)"=w302) -> ("error out"=w305:errorcluster)  [unwired: 5 in, 1 out]
        n161 = call-poly <vilib>:"Create Modbus Instance.vi"("error in"=w305, "port (502)"=u16 3) -> ("error out"=w306:errorcluster, "TCP slave instance"=w307:refnum<class "Modbus Slave.lvclass">)  [unwired: 8 in]
        n162 = case shown="无错误" w306 {
          tunnel: w310 -> [_ w312]
          tunnel: [enum16{"open", "read", "write", "close"}."write" w312] -> w309
          frame No Error {
          }
          frame Error {
          }
        }
      }
      frame "read" {
        n163 = case shown="无错误" w314 {
          tunnel: [enum16{"open", "read", "write", "close"}."write" enum16{"open", "read", "write", "close"}."close"] -> w315
          frame No Error {
          }
          frame Error {
          }
        }
      }
      frame "write" {
        n164 = local read "总氮测量数据区"() -> (w320:u16[])
        n165 = call-dynamic "Write Multiple Holding Registers.vi"("error in"=w326, "registers to write"=w320, "starting address"=u16 4096, "Modbus slave in"=w327) -> ("error out"=w323:errorcluster, "Modbus slave out"=w324:refnum<class "Modbus Slave.lvclass">)  [unwired: 6 in]
        n166 = local read "总氮状态告警区"() -> (w318:u16[])
        n167 = call-dynamic "Write Multiple Holding Registers.vi"("error in"=w323, "registers to write"=w318, "starting address"=u16 4224, "Modbus slave in"=w324) -> ("error out"=w321:errorcluster, "Modbus slave out"=w322:refnum<class "Modbus Slave.lvclass">)  [unwired: 6 in]
        n168 = case shown="无错误" w321 {
          tunnel: [enum16{"open", "read", "write", "close"}."write" enum16{"open", "read", "write", "close"}."close"] -> w328
          frame No Error {
          }
          frame Error {
          }
        }
      }
      frame "close" {
        n169 = call-dynamic "Shutdown.vi"("error in"=w332, "Modbus slave in"=w333) -> ("error out"=w331:errorcluster)  [unwired: 9 in]
        n170 = call <vilib>:"Clear Errors.vi"("error in (no error)"=w331) -> ("error out"=w335:errorcluster)  [unwired: 5 in, 1 out]
      }
    }
  }
